vi "trajectory_new_code_24_nov.vi"() -> ()   [LabVIEW 2019]
uses:
  <vilib>/FPGAPlugInAG/sbRIO-9629/niLvFpga_Open_sbRIO-9629.vi
  <vilib>/rvi/interface/common/dynamic/niFpgaDynamicAddResources.vi
  <vilib>/Utility/error.llb/Error Cluster From Error Code.vi
  <vilib>/rvi/errors/niLvFpgaAdjustHostInterfaceError.vi
  <vilib>/FPGAPlugInAG/Dynamic/niLvFpga_Close_Dynamic.vi
  <vilib>/rvi/interface/nirviOpenFPGA/nirviOpenFPGA.xnode
  FPGA Bitfiles/fcmsinglesection_FPGATarget_CloseLoopMotorTu_eGt+d+EV+VE.lvbitx
  Close_Loop_Motor_Tune.vi
  <vilib>/rvi/interface/nirviReadWriteControl/nirviReadWriteControl.xnode
  <vilib>/rvi/interface/nirviCloseFPGA/nirviCloseFPGA.xnode
  NiFpgaLv.dll
  <vilib>/rvi/interface/Simulation/niFpgaSimulationCallBeginRW.vi
panel:
  out "Desired Tip Position":dbl[](array[numeric])
  out "Numeric 2":i32
  out "theta3":dbl(graph)
  out "theta2":dbl(graph)
  out "theta1":dbl(graph)
  out "L_v":dbl
  out "alpha":dbl
  in  "Kp":dbl[](array[numeric])
  out "Error":bool
  in  "lower limit":dbl[](array[numeric])
  in  "upper limit":dbl[](array[numeric])
  out "error":dbl[](array[numeric])
  out "Current Tip Position":dbl[](array[numeric])
  out "Numeric":i32
  in  "radius":dbl=0.2
  in  "Degree Steps":dbl
  out "data out":string
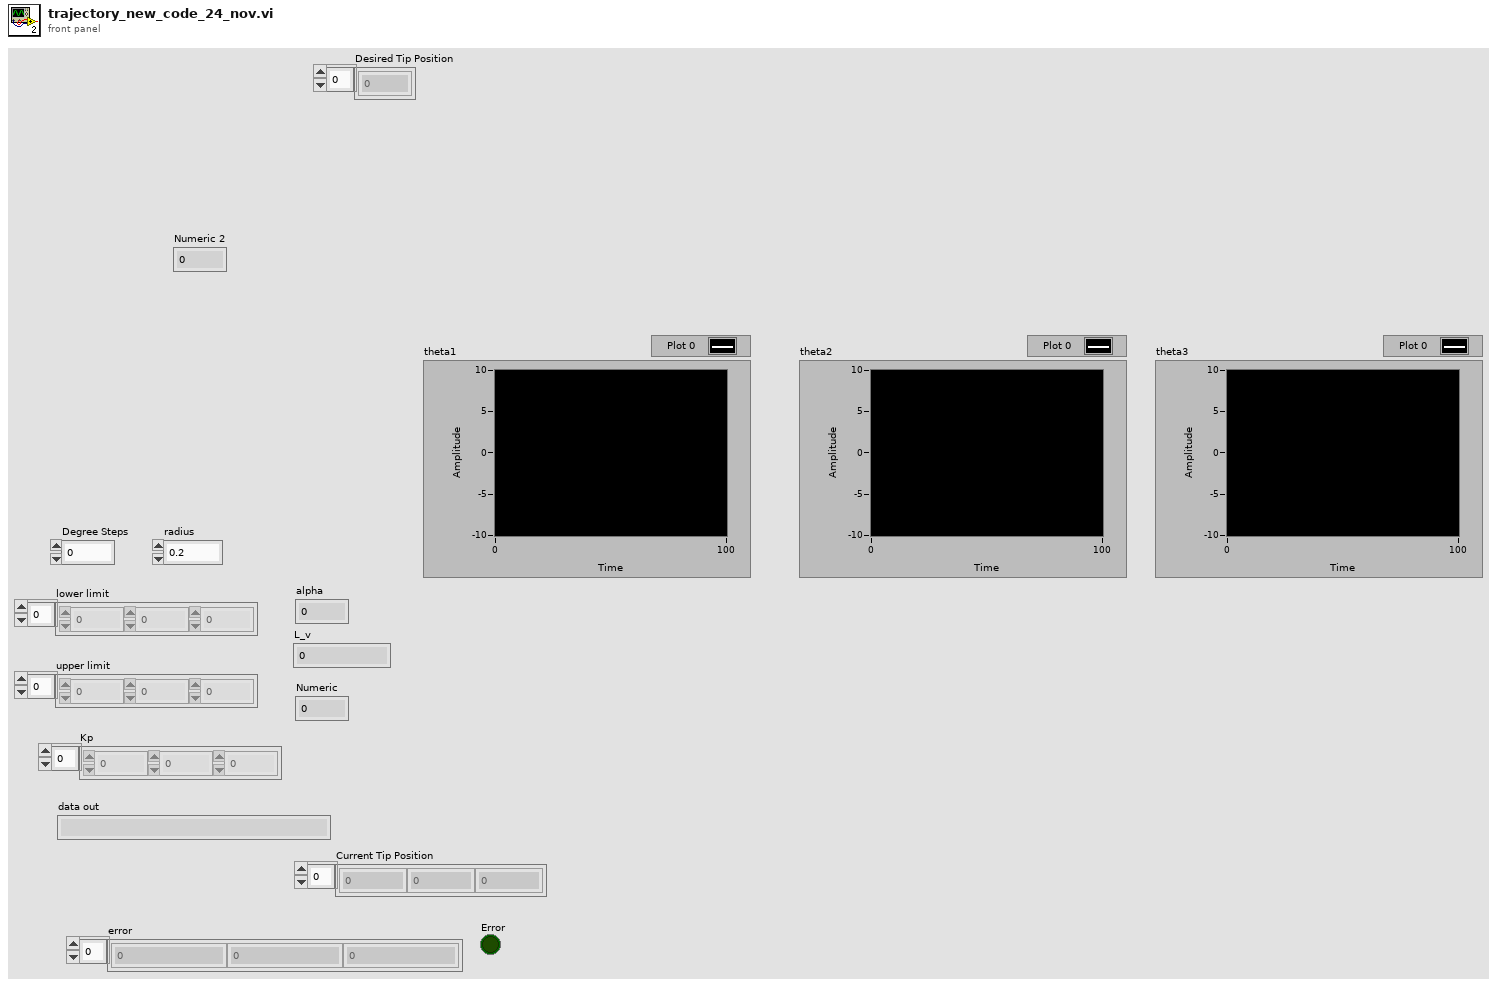
[diagram p1: front panel]
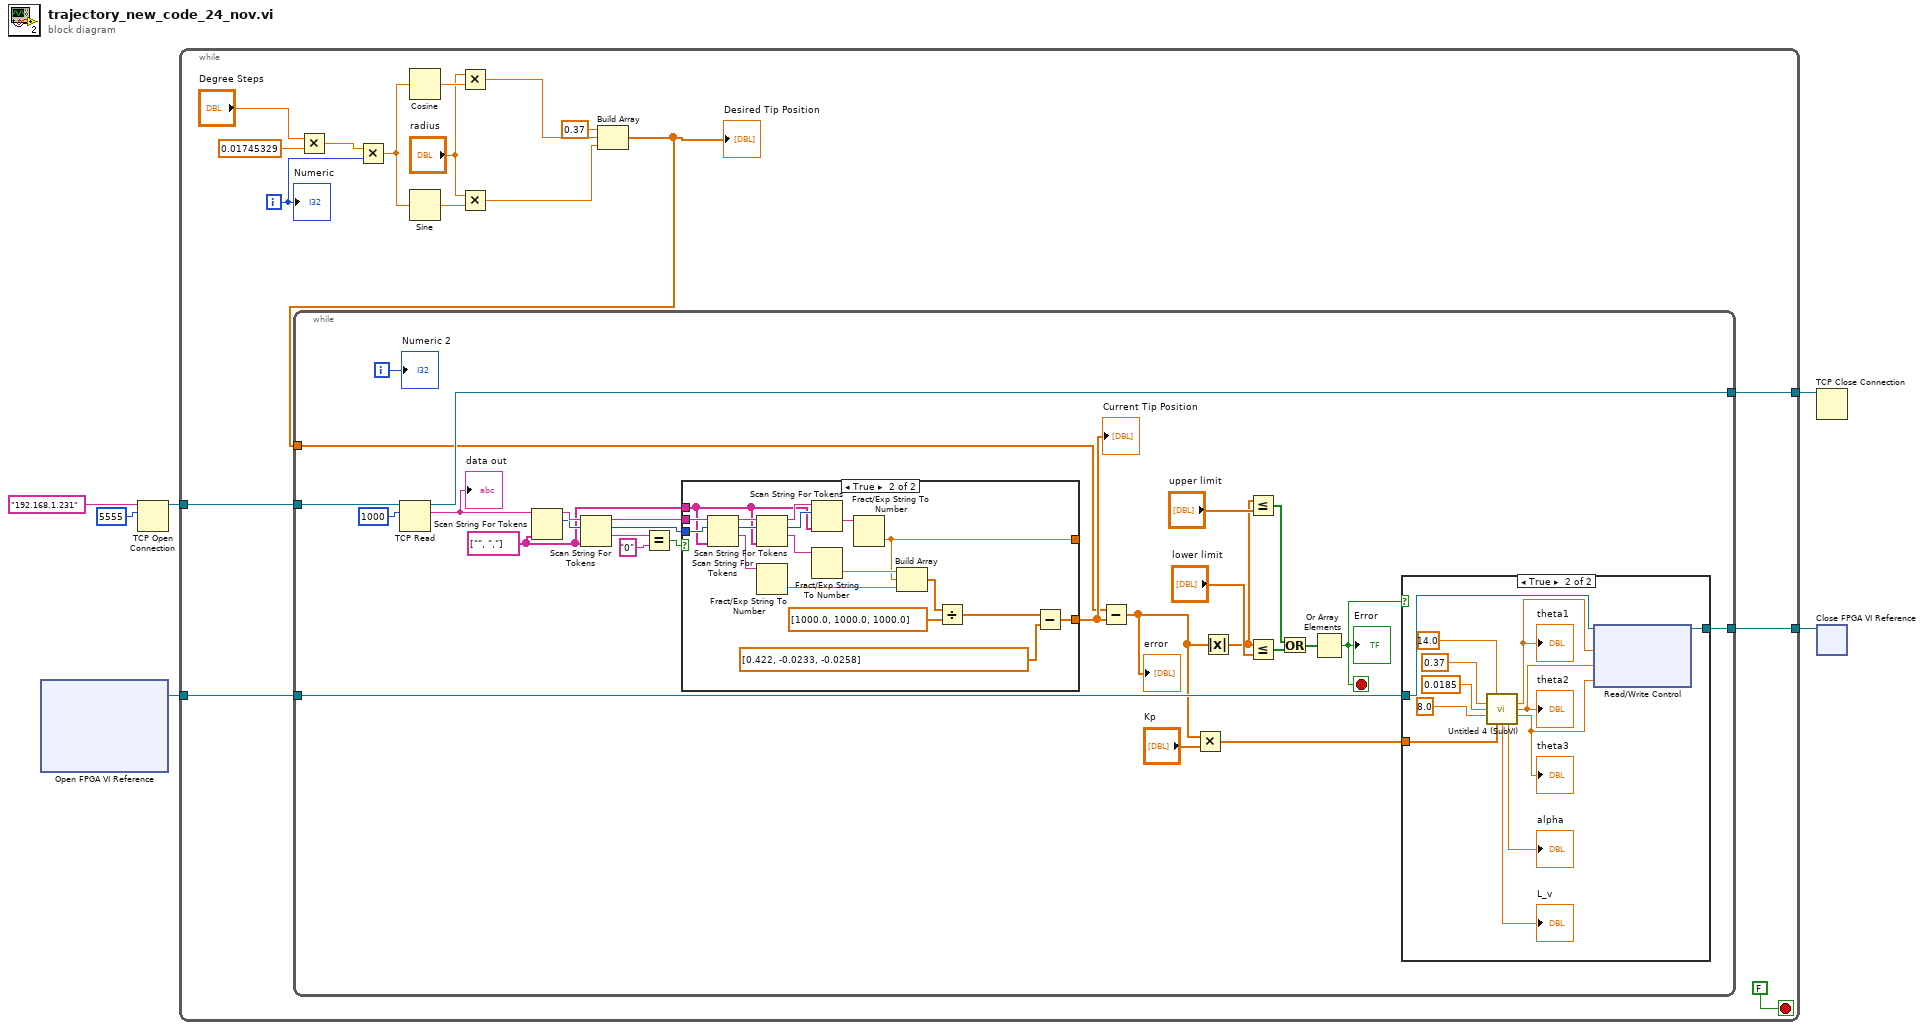
[diagram p0: block diagram]
diagram:
  n1 = xnode "Open FPGA VI Reference"() -> ("FPGA VI Reference Out"=w1:refnum<k20>)  [unwired: 2 in, 1 out]
  n2 = TCP Open Connection(address="192.168.1.231", remote port or service name=u16 5555) -> (connection ID=w6:refnum<k5>)  [unwired: 3 in, 1 out]
  n3 = while {
    tunnel: w6 -> [w23]
    tunnel: [w22] -> w5
    tunnel: [w12] -> w2
    tunnel: w1 -> [w11]
    i -> [w13]
    stop <- FALSE stop-if-true
    n4 = Multiply(x="Degree Steps", y=0.01745329) -> (x*y=w15:dbl)
    n5 = Multiply(x=w15, y=w13) -> (x*y=w18:dbl)
    n6 = Cosine(x=w18) -> (cos(x)=w20:dbl)
    n7 = Sine(x=w18) -> (sin(x)=w19:dbl)
    n8 = Multiply(x="radius", y=w20) -> (x*y=w10:dbl)
    n9 = Multiply(x="radius", y=w19) -> (x*y=w9:dbl)
    n10 = Build Array(0.37 ("element"), w10, w9) -> (w7:dbl[])
    "Desired Tip Position" <- w7
    n11 = while {
      tunnel: w23 -> [w50]
      tunnel: [w49] -> w22
      tunnel: w7 -> [w30]
      tunnel: [w28] -> w12
      tunnel: w11 -> [w27]
      i -> [w26]
      stop <- w25 stop-if-true
      w41 = string[] ["", ","] ("delimiters (\\s,\\t,\\r,\\n)")
      n12 = TCP Read(connection ID=w50, bytes to read=1000) -> (connection ID out=w49:refnum<k5>, data out=w43:string)  [unwired: 3 in, 1 out]
      "data out" <- w43
      n13 = Scan String For Tokens(6:w41, 9:w43) -> (2:w45:i32, 3:w46:string)  [unwired: 4 in, 2 out]
      n14 = Scan String For Tokens(6:w41, 8:w45, 9:w46) -> (1:w47:string, 2:w42:i32, 3:w40:string)  [unwired: 3 in, 1 out]
      n15 = Equal?(x=w47, y="0") -> (x = y?=w39:bool)
      n16 = case shown="True" w39 {
        tunnel: [_ w68] -> _
        tunnel: w40 -> [_ w64]
        tunnel: w42 -> [_ w66]
        tunnel: w41 -> [_ w63]
        tunnel: [_ w65] -> w38
        frame False {
        }
        frame True {
          n17 = Scan String For Tokens(6:w63, 8:w66, 9:w64) -> (1:w76:string, 2:w78:i32, 3:w80:string)  [unwired: 3 in, 1 out]
          n18 = Scan String For Tokens(6:w63, 8:w78, 9:w80) -> (1:w75:string, 2:w77:i32, 3:w79:string)  [unwired: 3 in, 1 out]
          n19 = Fract/Exp String To Number(string=w76) -> (number=w67:dbl)  [unwired: 3 in, 1 out]
          n20 = Scan String For Tokens(6:w63, 8:w77, 9:w79) -> (1:w74:string)  [unwired: 3 in, 3 out]
          n21 = Fract/Exp String To Number(string=w75) -> (number=w69:dbl)  [unwired: 3 in, 1 out]
          n22 = Fract/Exp String To Number(string=w74) -> (number=w68:dbl)  [unwired: 3 in, 1 out]
          n23 = Build Array(w69, w68, w67) -> (w73:dbl[])
          n24 = Divide(x=w73, y=dbl[] [1000.0, 1000.0, 1000.0]) -> (x/y=w71:dbl[])
          n25 = Subtract(x=w71, y=dbl[] [0.422, -0.0233, -0.0258]) -> (x-y=w65:dbl[])
        }
      }
      "Current Tip Position" <- w38
      n26 = Subtract(x=w30, y=w38) -> (x-y=w24:dbl[])
      "error" <- w24
      n27 = Multiply(x=w24, y="Kp") -> (x*y=w29:dbl[])
      n28 = Absolute Value(x=w24) -> (abs(x)=w32:dbl[])
      n29 = Less Or Equal?(x=w32, y="upper limit") -> (x <= y?=w35:bool[])
      n30 = Less Or Equal?(x=w32, y="lower limit") -> (x <= y?=w34:bool[])
      n31 = Or(x=w35, y=w34) -> (x .or. y?=w33:bool[])
      n32 = Or Array Elements(Boolean array=w33) -> (logical OR=w25:bool)
      "Error" <- w25
      n33 = case shown="True" w25 {
        tunnel: w29 -> [_ w62]
        tunnel: [_ w55] -> w28
        tunnel: w27 -> [_ w51]
        frame False {
        }
        frame True {
          n34 = call "Untitled 4 (SubVI).vi"("Radius of motor pulley\n (mm)"=14.0 ("Radius of motor pulley\n (mm)"), "Length of the FCM (m)"=0.37, "Radius of disk (m)"=0.0185, "Number of Disks"=8.0, "Tip position Input"=w62) -> ("theta1"=w54:dbl, "theta2"=w53:dbl, "theta3"=w52:dbl, "L_v"=→"L_v":dbl, "alpha"=→"alpha":dbl)  [unwired: 2 in, 4 out]
          "theta1" <- w54
          "theta2" <- w53
          "theta3" <- w52
          n35 = xnode "Read/Write Control"("FPGA VI Reference In"=w51, "desired angle"=w54, "desired angle 2"=w53, "desired angle 3"=w52) -> ("FPGA VI Reference Out"=w55:refnum<k20>)  [unwired: 1 in, 1 out]
        }
      }
      "Numeric 2" <- w26
    }
    "Numeric" <- w13
  }
  n36 = TCP Close Connection(connection ID=w5) -> ()  [unwired: 2 in, 2 out]
  n37 = xnode "Close FPGA VI Reference"("FPGA VI Reference In"=w2) -> ()  [unwired: 1 in, 1 out]
